vi "Send Shutdown Command.vi"(8 "error in (no error)":errorcluster, 11 "Plugin Interface in":refnum<class "Plugin Interface.lvclass">) -> (0 "error out":errorcluster, 3 "Plugin Interface out":refnum<class "Plugin Interface.lvclass">)   [LabVIEW 2017, in "DSF Core.lvlib" / "Plugin Interface.lvclass"]
uses:
  Interfaces/Transceiver Interface/Plugin Interface.lvclass
  C:/Git/DSF/Data Sharing Framework/Source/Core/Engine/Classes/Interfaces/Interface/Interface.lvclass
  Interfaces/Transceiver Interface/Command Data.ctl
  Interfaces/Transceiver Interface/Command.ctl
  Interfaces/Transceiver Interface/Command Parameters.ctl
  Interfaces/Interface/Interface.lvclass/Interface.ctl
  Interfaces/Transceiver Interface/Response.ctl
  Interfaces/Transceiver Interface/Write Plugin Command.vi
  Interfaces/Interface/Write Command.vi
  Interfaces/Interface/Write RT FIFO.vi
  Interfaces/Dispatcher/Command Timeout.vi
  Interfaces/Transceiver Interface/Read Plugin Response.vi
  Interfaces/Dispatcher/Invalid Response.vi
  Interfaces/Interface/Interface.lvclass
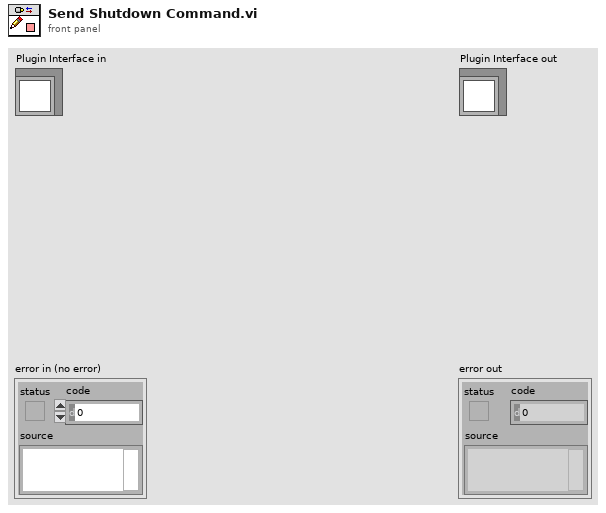
[diagram p1: front panel]
types:
  T1 = typedef "DSF Core.lvlib/Plugin Interface.lvclass/Command Data.ctl" = cluster{"Command":T2, "Parameters":T3}
  T2 = typedef "DSF Core.lvlib/Plugin Interface.lvclass/Command.ctl" = enum8{"Set Inline Buffer", "Rx", "Tx", "Shutdown"}
  T3 = typedef "DSF Core.lvlib/Plugin Interface.lvclass/Command Parameters.ctl" = cluster{"arg1":u64, "arg2":u64}
  T4 = typedef "DSF Core.lvlib/Plugin Interface.lvclass/Response.ctl" = enum8{"General Ack", "Shutting Down"}
  T5 = typedef "DSF Core.lvlib/Plugin Interface.lvclass/Response Data.ctl" = cluster{"Response":T4, "Parameters":T6}
  T6 = typedef "DSF Core.lvlib/Plugin Interface.lvclass/Response Parameters.ctl" = cluster{"arg1":u64, "arg2":u64}
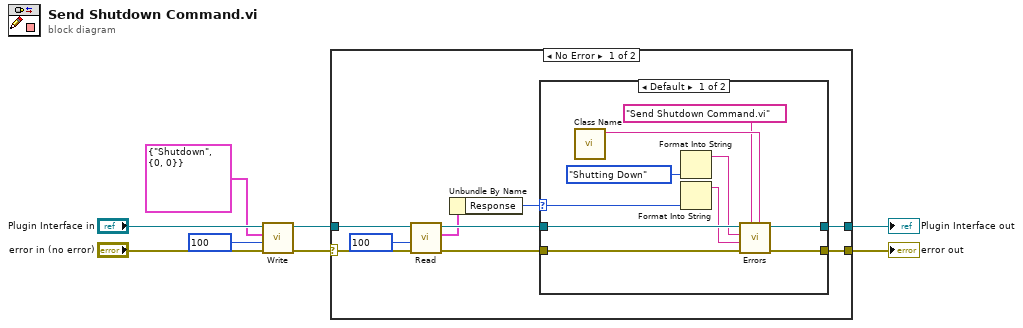
[diagram p0: block diagram]
diagram:
  n1 = call-poly "Write.vi"("error in (no error)"="error in (no error)", "timeout in ms (0)"=100, "command"=T1 {"Command"=enum."Shutdown", "Parameters"={"arg1"=0, "arg2"=0}}, "Plugin Interface in"="Plugin Interface in") -> ("error out"=w4:errorcluster, "Plugin Interface out"=w5:refnum<class "Plugin Interface.lvclass">)  [unwired: 6 in]
  n2 = case shown="No Error" w4 {
    selector: w4 -> [w11 w30]
    tunnel: w5 -> [w14 w31]
    tunnel: [w17 w30] -> w8
    tunnel: [w16 w31] -> w7
    frame No Error {
      n3 = call-poly "Read.vi"("error in (no error)"=w11, "timeout in ms (0)"=100, "Plugin Interface in"=w14) -> ("error out"=w12:errorcluster, "response"=w9:T5, "Plugin Interface out"=w13:refnum<class "Plugin Interface.lvclass">)  [unwired: 5 in, 1 out]
      n4 = Unbundle By Name(w9) -> ("Response"=w15:T4)
      n5 = case shown="Default" w15 {
        selector: w15 -> [w21 _]
        tunnel: w12 -> [w26 w29]
        tunnel: [w24 w29] -> w17
        tunnel: w13 -> [w27 w28]
        tunnel: [w25 w28] -> w16
        frame Default {
          n6 = call "Class Name.vi"() -> ("class name"=w19:string)  [unwired: 11 in]
          n7 = Format Into String(Response."Shutting Down" ("x")) -> (resulting string=w22:string)  [unwired: 3 in, 1 out]
          n8 = Format Into String(w21) -> (resulting string=w20:string)  [unwired: 3 in, 1 out]
          n9 = call-poly "Errors.vi"("error source class name"=w19, "error source vi name"="Send Shutdown Command.vi", "error in (no error)"=w26, "actual response"=w20, "expected response"=w22, "Interface in"=w27) -> ("error out"=w24:errorcluster, "Interface out"=w25:refnum<class "Plugin Interface.lvclass">)  [unwired: 4 in]
        }
        frame "Shutting Down" {
        }
      }
    }
    frame Error {
    }
  }
  "error out" <- w8
  "Plugin Interface out" <- w7
